vi "CleanUp.vi"(0 "object in":refnum<class "Hamamatsu.lvclass">, 5 "error in (no error)":errorcluster) -> (14 "object out":refnum<class "Hamamatsu.lvclass">, 19 "error out":errorcluster)   [LabVIEW 2021, in "Hamamatsu.lvclass"]
uses:
  Hamamatsu.lvclass
  Hamamatsu.lvclass/Hamamatsu.ctl
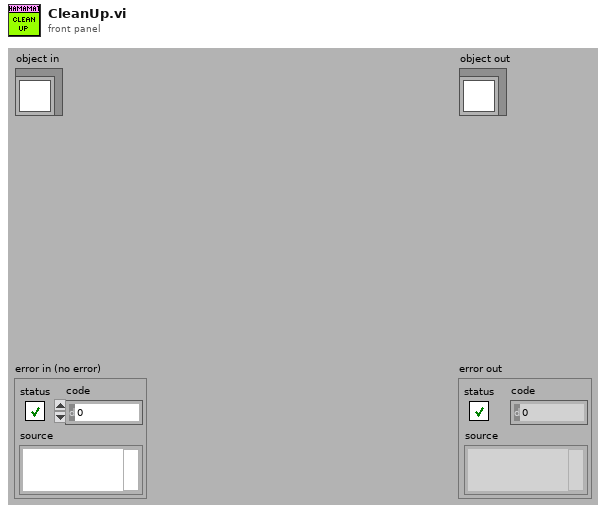
[diagram p1: front panel]
types:
  T1 = typedef "IMAQ Image.ctl" = refnum<image>
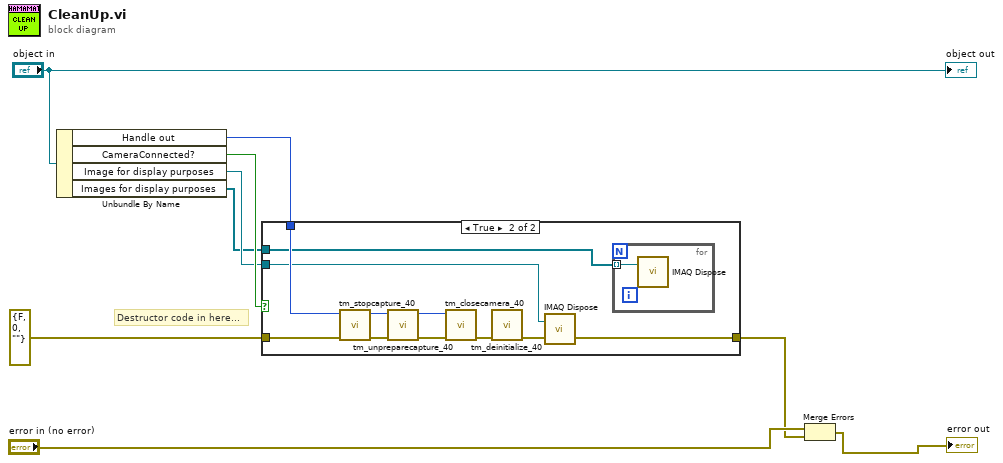
[diagram p0: block diagram]
diagram:
  # "Destructor code in here..."
  n1 = Unbundle By Name("object in") -> ("Handle out"=w6:u32, "CameraConnected?"=w3:bool, "Image for display purposes"=w2:T1, "Images for display purposes"=w1:T1[])
  n2 = case shown="True" w3 {
    tunnel: w6 -> [_ w15]
    tunnel: errorcluster {"status"=FALSE, "code"=0, "source"=""} ("error in (no error)") -> [w10 w17]
    tunnel: [w10 w12] -> w4
    tunnel: w2 -> [_ w14]
    tunnel: w1 -> [_ w11]
    frame False {
    }
    frame True {
      n3 = call <userlib>:"tm_stopcapture_40.vi"("error in (no error)"=w17, "Handle in"=w15) -> ("error out"=w19:errorcluster, "Handle out"=w20:u32)  [unwired: 8 in]
      n4 = call <userlib>:"tm_unpreparecapture_40.vi"("error in (no error)"=w19, "Handle in"=w20) -> ("error out"=w18:errorcluster, "Handle out"=w16:u32)  [unwired: 8 in]
      n5 = call <userlib>:"tm_closecamera_40.vi"("error in (no error)"=w18, "Handle in"=w16) -> ("error out"=w21:errorcluster)  [unwired: 9 in]
      n6 = call <userlib>:"tm_deinitialize_40.vi"("error in (no error)"=w21) -> ("error out"=w13:errorcluster)  [unwired: 10 in]
      n7 = call "IMAQ Dispose"("Image"=w14, "error in (no error)"=w13) -> ("error out"=w12:errorcluster)  [unwired: 4 in]
      n8 = for {
        tunnel: w11 -> [w22] mode=indexing
        n9 = call "IMAQ Dispose"("Image"=w22) -> ()  [unwired: 5 in, 1 out]
      }
    }
  }
  n10 = Merge Errors("error in (no error)", w4) -> (→"error out":errorcluster)
  "object out" <- "object in"
